vi "Highlight Execution And Prob Data.vi"() -> ()   [LabVIEW 2012]
panel:
  in  "Switch":bool caption="Boolean"
  out "Gauge":dbl(knob) scale=0.0..2000.0
  # "Ounces"
  # "Grams"
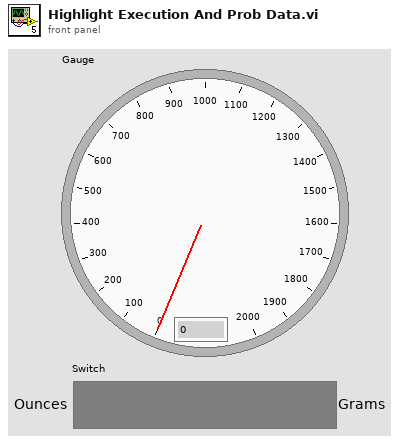
[diagram p1: front panel]
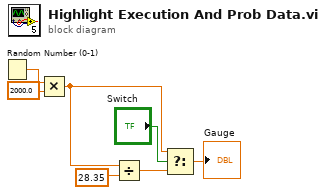
[diagram p0: block diagram]
diagram:
  n1 = Random Number (0-1) ("Random Number (0-2000)")() -> (number: 0 to 1=w6:dbl)
  n2 = Multiply(x=w6, y=2000.0) -> (x*y=w2:dbl)
  n3 = Divide(x=w2, y=28.35) -> (x/y=w1:dbl)
  n4 = Select(t=w2, s="Switch", f=w1) -> (s? t:f=→"Gauge":dbl)
